vi "Write.vi"(8 "error in (no error)":errorcluster, 10 "DATA":T1, 11 "Notifiers in":refnum<class "Notifiers.lvclass">) -> (0 "error out":errorcluster, 3 "Notifiers out":refnum<class "Notifiers.lvclass">)   [LabVIEW 2020, in "Notifiers.lvclass"]
uses:
  Notifiers.lvclass
  Notifiers.lvclass/Notifiers.ctl
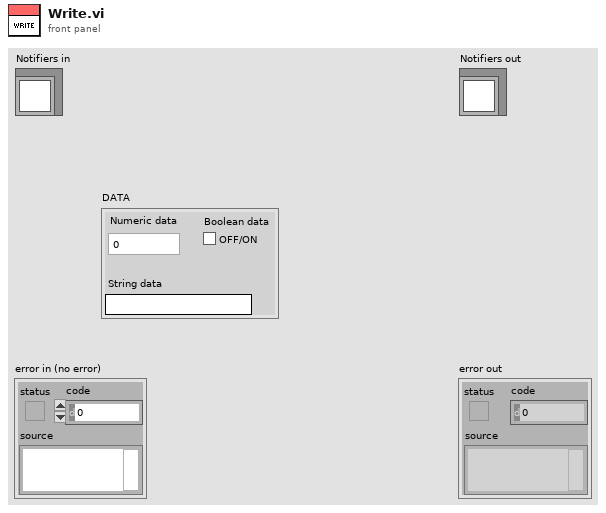
[diagram p1: front panel]
types:
  T1 = cluster{"Numeric data":dbl, "String data":string, "Boolean data":bool}
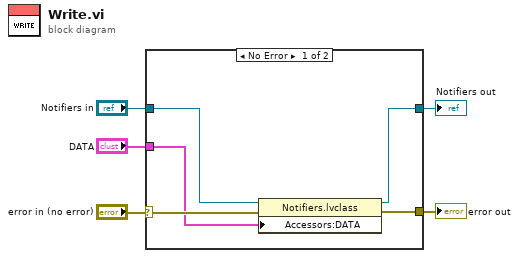
[diagram p0: block diagram]
diagram:
  n1 = case shown="No Error" "error in (no error)" {
    selector: "error in (no error)" -> [w10 w12]
    tunnel: [w9 w12] -> w4
    tunnel: [w7 w11] -> w2
    tunnel: "Notifiers in" -> [w8 w11]
    tunnel: "DATA" -> [w6 _]
    frame No Error {
      n2 = property class="Notifiers.lvclass"(reference=w8, error in=w10, "Accessors:DATA"=w6) -> (reference out=w7:refnum<class "Notifiers.lvclass">, error out=w9:errorcluster)
    }
    frame Error {
    }
  }
  "error out" <- w4
  "Notifiers out" <- w2
